vi "TCP-IP Mgr.Create.vi"(6 "Status_Rcv Q Items":T1={"Status.Q.Msg"={"Cmd"="Task", "Sub"="TCP-IP Connect Event", "Data1"=variant, "Data2"=variant}, "Rcv.Q.Msg"={"Cmd"="Task", "Sub"="TCP-IP Rcv", "Data1"=variant, "Data2"=variant}}, 7 "Index":i32, 8 "Error In":errorcluster, 9 "Config":T3={"IP"="127.0.0.1", "Port"=8500, "Listener"=FALSE, "Enable"=FALSE}, 10 "Q Name":string="TCP-IP Mgr", 11 "Parent Q":refnum<queue>) -> (0 "Error Out":errorcluster, 2 "Name Out":string, 3 "reference out":refnum<vi>)   [LabVIEW 2024, in "EQMF.lvlib" / "TCP-IP.lvlib"]
uses:
  TCP-IP.lvlib
  Queues/Q.Element.ctl
  TCP-IP Mgr.Config.ctl
  TCP-IP Mgr.Cluster - Q Message Templates.ctl
  _Core/TCP-IP Mgr.Core.vi
  Module/Module Utils.lvlib
  Queues/Queue Utils.lvlib
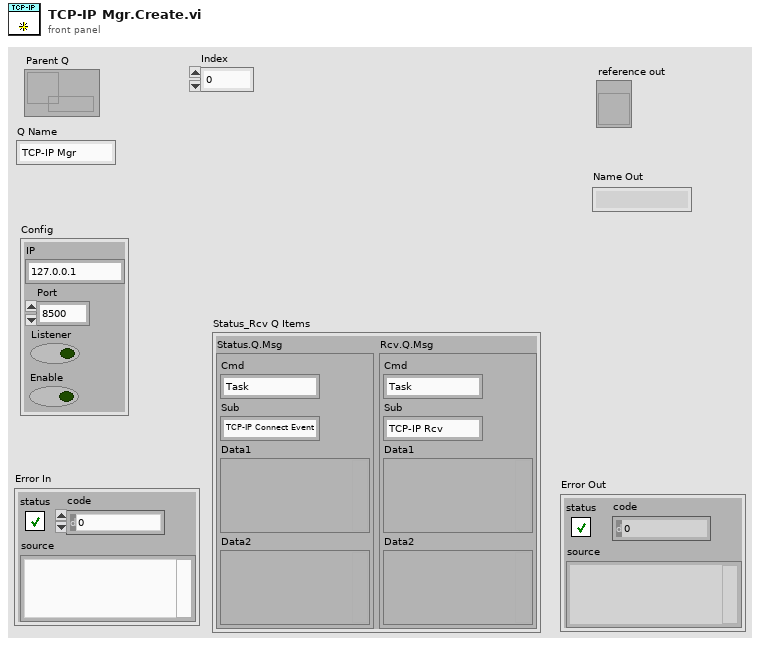
[diagram p1: front panel]
types:
  T1 = typedef "EQMF.lvlib/TCP-IP.lvlib/TCP-IP Mgr.Cluster - Q Message Templates.ctl" = cluster{"Status.Q.Msg":T2, "Rcv.Q.Msg":T2}
  T2 = typedef "EQMF.lvlib/Queue Utils.lvlib/Q.Element.ctl" = cluster{"Cmd":string, "Sub":string, "Data1":variant, "Data2":variant}
  T3 = typedef "EQMF.lvlib/TCP-IP.lvlib/TCP-IP Mgr.Config.ctl" = cluster{"IP":string, "Port":u16, "Listener":bool, "Enable":bool}
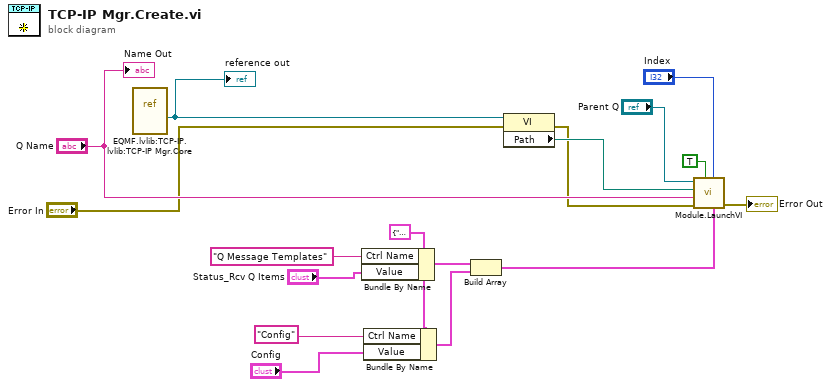
[diagram p0: block diagram]
diagram:
  w4 = cluster{"Ctrl Name":string, "Value":variant} {"Ctrl Name"="", "Value"=variant} ("Cluster")
  n1 = vi-ref "EQMF.lvlib:TCP-IP.lvlib:TCP-IP Mgr.Core.vi"() -> (w10:refnum<vi>)
  "reference out" <- w10
  n2 = Bundle By Name(cluster=w4, "Ctrl Name"="Q Message Templates", "Value"="Status_Rcv Q Items") -> (w3:cluster{"Ctrl Name":string, "Value":variant})
  n3 = Bundle By Name(cluster=w4, "Ctrl Name"="Config", "Value"="Config") -> (w2:cluster{"Ctrl Name":string, "Value":variant})
  n4 = Build Array(w3, w2) -> (w1:cluster{"Ctrl Name":string, "Value":variant}[])
  n5 = property class="VI"(reference=w10, error in="Error In") -> (error out=w11:errorcluster, "Path"=w12:path)  [unwired: 1 out]
  n6 = call "Module.LaunchVI.vi"("Init Ctrl Values"=w1, "Index"="Index", "Reentrant"=TRUE, "error in"=w11, "Q Name"="Q Name", "VI Path"=w12, "Parent Q"="Parent Q") -> ("error out"=→"Error Out":errorcluster)  [unwired: 2 in, 2 out]
  "Name Out" <- "Q Name"
